vi "FWHM X and Y Graph.vi"(1 "Input Arrays":cluster{"X-array":dbl[], "Y-array":dbl[]} {"Y-array" format="%.2f"; "X-array" format="%.2f"}) -> (0 "FWHM":dbl format="%.2f")   [LabVIEW 2023]
uses:
  <vilib>/Analysis/NI_AALPro.lvlib
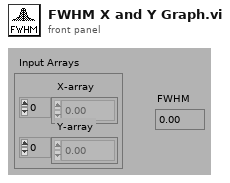
[diagram p1: front panel]
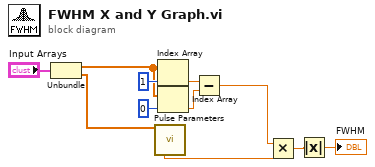
[diagram p0: block diagram]
diagram:
  n1 = Unbundle("Input Arrays") -> ("X-array"=w5:dbl[], "Y-array"=w4:dbl[])
  n2 = call <vilib>:"Pulse Parameters.vi"("X"=w4) -> ("duration"=w6:dbl)  [unwired: 4 in, 10 out]
  n3 = Index Array(array=w5, index=1 ("Index")) -> (element=w7:dbl)
  n4 = Index Array(array=w5, index=0 ("Index")) -> (element=w8:dbl)
  n5 = Subtract(x=w7, y=w8) -> (x-y=w3:dbl)
  n6 = Multiply(x=w3, y=w6) -> (x*y=w2:dbl)
  n7 = Absolute Value(x=w2) -> (abs(x)=→"FWHM":dbl)
